vi "AB_API Set Destination.vi"(8 "error in (no error)":errorcluster, 9 "source item ID":string, 10 "Destination label":string, 11 "Build in":refnum<class "AB_Build.lvclass">) -> (0 "error out":errorcluster, 3 "Build out":refnum<class "AB_Build.lvclass">)   [LabVIEW 2020]
uses:
  <vilib>/AppBuilder/AB_Classes/Build/AB_Build.lvclass
  <vilib>/AppBuilder/AB_API/common/AB_API Apply Setting Type.ctl
  <vilib>/AppBuilder/AB_Classes/Source/AB_Source.lvclass
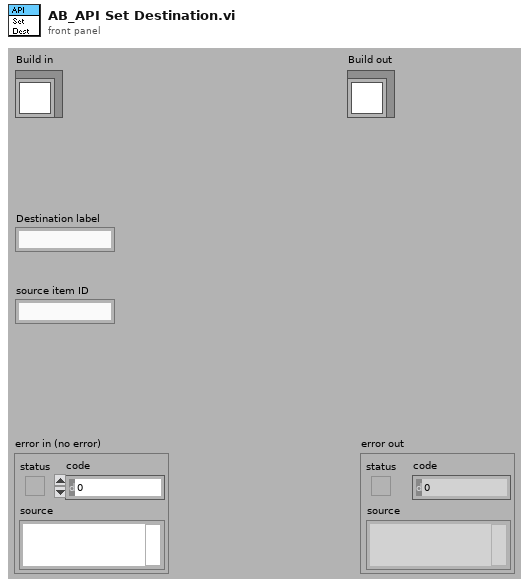
[diagram p1: front panel]
types:
  T1 = typedef "AB_API Apply Setting Type.ctl" = enum16{"Inclusion", "Destination", "Properties", "Password", "Prefix", "SaveSettings"}
  T2 = typedef "AB_Build.ctl" = cluster{"buildSpecName":string, "buildSpecDescription":string, "destinations":refnum<class "AB_Destination.lvclass">[], "exclusionOption":T3, "defaultLanguage":string, "supportedLanguages":string[], "excludedDirectories":path[], "buildContext":refnum<vi>, "buildObject":T4, "preview":bool, "programatic":bool, "progressBarEvents":T5, "userLog_Path":path, "preActionID":string, "preAction_Path":path, "postActionID":string, "postAction_Path":path, "eng_checkForBrokenVIs?":bool, "eng_verboseLinkerErrors?":bool, "localDest_Path":path, "targetDest_Path":path, "removeVIObject":u16, "cache":refnum<class "PreviewCache.lvclass">, "use cache":bool, "previewCache_ID":string, "buildCache_ID":string, "eng_TempLocalDest_Path":path, "eng_collectDependencies?":bool, "versionInfo":cluster{"buildVersion":cluster{"major":u16, "minor":u16, "patch":u16, "build":u16}, "autoIncrement":bool}, "eng_enableVIChecksums":bool}
  T3 = typedef "AB_Exclusion_Option.ctl" = cluster{"typedefs":bool, "polymorphicVIs":bool, "unusedLibraryItems":bool, "modifyLibraryFile":bool, "edit-timeDependencies":bool, "inlineVIs":bool, "dependent PPLs":bool, "dependent DLLs":bool}
  T4 = typedef "ItemRef.ctl" = u64
  T5 = typedef "provcom_ProgressBar_Events.ctl" = cluster{"newJob":refnum<user-event>, "newItem":refnum<user-event>, "errorMsg":T6, "cancel":refnum<user-event>}
  T6 = typedef "mxLvBuildError.ctl" = refnum<user-event>
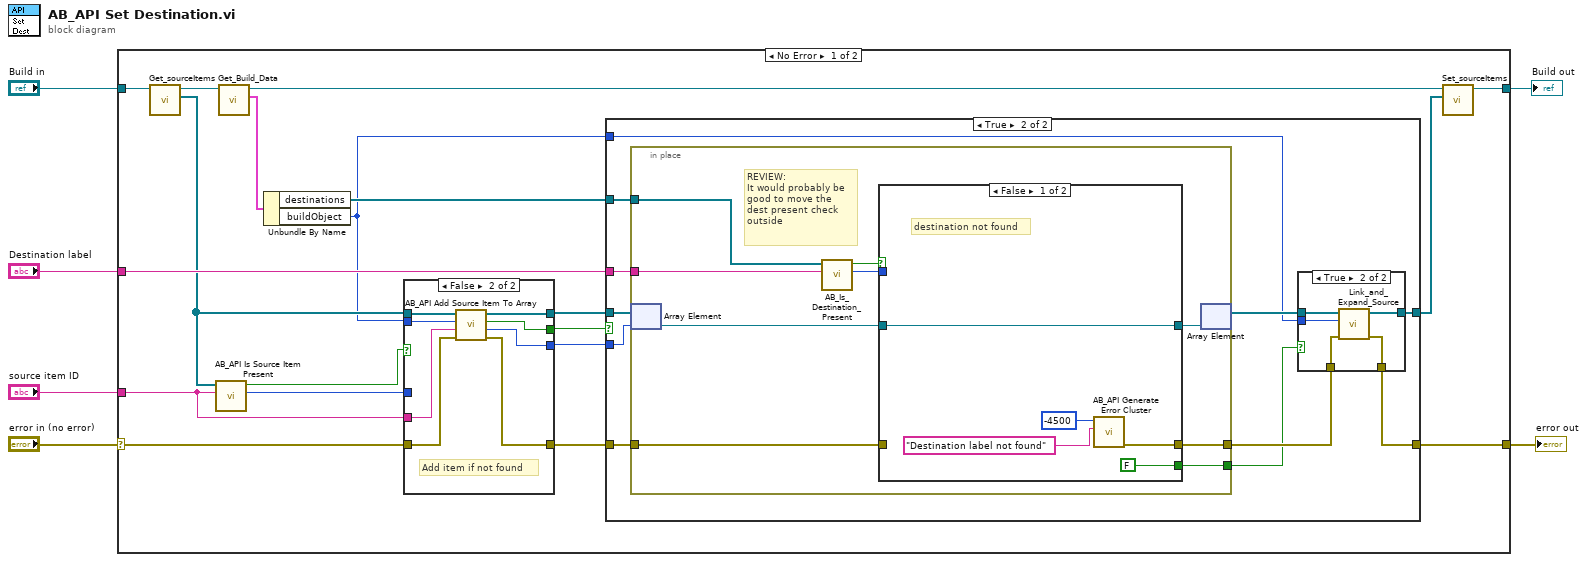
[diagram p0: block diagram]
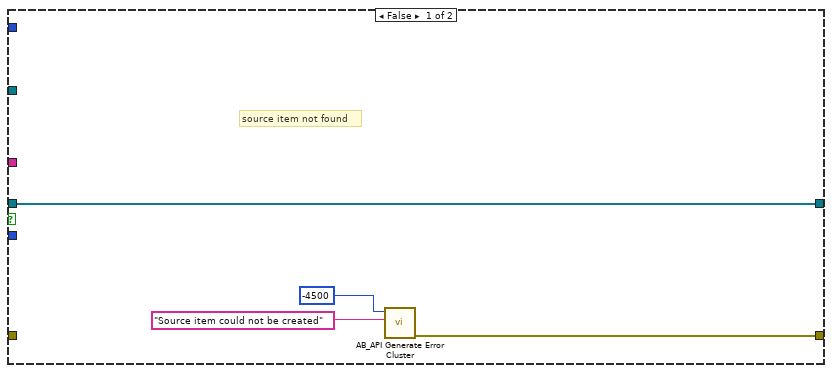
[diagram p3: hidden frame]
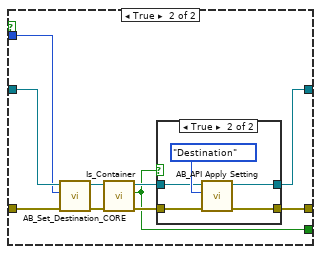
[diagram p5: hidden frame]
diagram:
  n1 = case shown="No Error" "error in (no error)" {
    selector: "error in (no error)" -> [w14 w92]
    tunnel: [w22 w92] -> w5
    tunnel: [w24 w91] -> w4
    tunnel: "Build in" -> [w23 w91]
    tunnel: "source item ID" -> [w12 _]
    tunnel: "Destination label" -> [w21 _]
    frame No Error {
      n2 = call <vilib>:"Get_sourceItems.vi"("Class in"=w23) -> ("sourceItems"=w16:refnum<class "AB_Source.lvclass">[], "Class out"=w20:refnum<class "AB_Build.lvclass">)  [unwired: 1 in, 8 out]
      n3 = call <vilib>:"AB_API Is Source Item Present.vi"("item ID"=w12, "source items"=w16) -> ("index"=w8:i32, "source item present?"=w11:bool)  [unwired: 1 in, 7 out]
      n4 = call <vilib>:"Get_Build_Data.vi"("Class in"=w20) -> ("data"=w18:T2, "Class out"=w19:refnum<class "AB_Build.lvclass">)  [unwired: 1 in, 8 out]
      n5 = Unbundle By Name(w18) -> ("destinations"=w17:refnum<class "AB_Destination.lvclass">[], "buildObject"=w7:T4)
      n6 = case shown="False" w11 {
        selector: w11 -> [w29 _]
        tunnel: [w29 w32] -> w10
        tunnel: [w28 w34] -> w13
        tunnel: w14 -> [w28 w35]
        tunnel: [w26 w33] -> w9
        tunnel: w12 -> [_ w31]
        tunnel: [w27 w36] -> w15
        tunnel: w16 -> [w27 w37]
        tunnel: w8 -> [w26 _]
        tunnel: w7 -> [_ w30]
        frame True {
        }
        frame False {
          # "Add item if not found"
          n7 = call <vilib>:"AB_API Add Source Item To Array.vi"("error in (no error)"=w35, "source item ID"=w31, "buildObject"=w30, "source items in"=w37) -> ("error out"=w34:errorcluster, "index"=w33:i32, "added?"=w32:bool, "source items out"=w36:refnum<class "AB_Source.lvclass">[])  [unwired: 4 in]
        }
      }
      n8 = case shown="True" w10 {
        tunnel: w21 -> [_ w52]
        tunnel: w9 -> [_ w51]
        tunnel: w15 -> [w41 w50]
        tunnel: [w41 w45] -> w25
        tunnel: w13 -> [_ w49]
        tunnel: [w38 w43] -> w22
        tunnel: w17 -> [_ w48]
        tunnel: w7 -> [_ w46]
        frame False {
          # "source item not found"
          n9 = call <vilib>:"AB_API Generate Error Cluster.vi"("Additional Message"="Source item could not be created", "Code"=-4500) -> ("error out"=w38:errorcluster)  [unwired: 2 in, 7 out]
        }
        frame True {
          n10 = in-place {
            in-place-border: w52 -> [w63]
            in-place-border: w49 -> [w66]
            in-place-border: [w67] -> w44
            in-place-border: w48 -> [w61]
            in-place-border: [w60] -> w42
            # "REVIEW:\nIt would probably be\ngood to move the \ndest present check \noutside"
            n11 = in-place-array #1(w50, w51) -> (w62:refnum<class "AB_Source.lvclass">)
            n12 = call <vilib>:"AB_Is_Destination_Present.vi"("destination label"=w63, "destinations"=w61) -> ("index"=w64:i32, "destination present?"=w65:bool)  [unwired: 1 in, 7 out]
            n13 = case shown="False" w65 {
              tunnel: w64 -> [_ w82]
              tunnel: [w70 w80] -> w68
              tunnel: [w71 w79] -> w67
              tunnel: w66 -> [_ w81]
              tunnel: w62 -> [w70 w83]
              tunnel: [FALSE ("container") w74] -> w60
              frame False {
                # "destination not found"
                n14 = call <vilib>:"AB_API Generate Error Cluster.vi"("Additional Message"="Destination label not found", "Code"=-4500) -> ("error out"=w71:errorcluster)  [unwired: 2 in, 7 out]
              }
              frame True {
                n15 = call <vilib>:"AB_Set_Destination_CORE.vi"("error in (no error)"=w81, "destination index"=w82, "Source in"=w83) -> ("error out"=w76:errorcluster, "Source out"=w78:refnum<class "AB_Source.lvclass">)  [unwired: 7 out]
                n16 = call-dynamic "Is_Container.vi"("error in (no error)"=w76, "AB_Source in"=w78) -> ("error out"=w75:errorcluster, "container"=w74:bool, "AB_Source out"=w77:refnum<class "AB_Source.lvclass">)  [unwired: 7 in]
                n17 = case shown="True" w74 {
                  tunnel: [w85 w90] -> w80
                  tunnel: [w84 w89] -> w79
                  tunnel: w77 -> [w85 w87]
                  tunnel: w75 -> [w84 w86]
                  frame False {
                  }
                  frame True {
                    n18 = call <vilib>:"AB_API Apply Setting.vi"("error in (no error)"=w86, "Settings"=AB_API_Apply_Setting_Type."Destination", "Source in"=w87) -> ("error out"=w89:errorcluster, "Source out"=w90:refnum<class "AB_Source.lvclass">)  [unwired: 7 in]
                  }
                }
              }
            }
            n19 = in-place-array #1(w68) -> (w47:refnum<class "AB_Source.lvclass">[])  [unwired: 1 out]
          }
          n20 = case shown="True" w42 {
            tunnel: w47 -> [w54 w59]
            tunnel: [w54 w58] -> w45
            tunnel: w46 -> [_ w57]
            tunnel: w44 -> [w53 w56]
            tunnel: [w53 w55] -> w43
            frame False {
            }
            frame True {
              n21 = call <vilib>:"Link_and_Expand_Source.vi"("error in (no error)"=w56, "Object"=w57, "AB_Source in"=w59) -> ("error out"=w55:errorcluster, "AB_Source out"=w58:refnum<class "AB_Source.lvclass">[])  [unwired: 7 in]
            }
          }
        }
      }
      n22 = call <vilib>:"Set_sourceItems.vi"("sourceItems"=w25, "Class in"=w19) -> ("Class out"=w24:refnum<class "AB_Build.lvclass">)  [unwired: 1 in, 8 out]
    }
    frame Error {
    }
  }
  "error out" <- w5
  "Build out" <- w4
